vi "CH3_Save_Header.vi"() -> ()   [LabVIEW 2018]
uses:
  RxTx/RxTx.lvclass
  Save Image/Save Image.lvclass
panel:
  in  "Save Image out":refnum<class "Save Image.lvclass">
  in  "RxTx.lvclass":refnum<class "RxTx.lvclass">
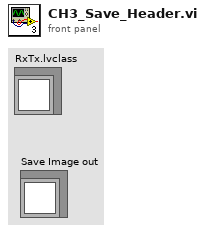
[diagram p1: front panel]
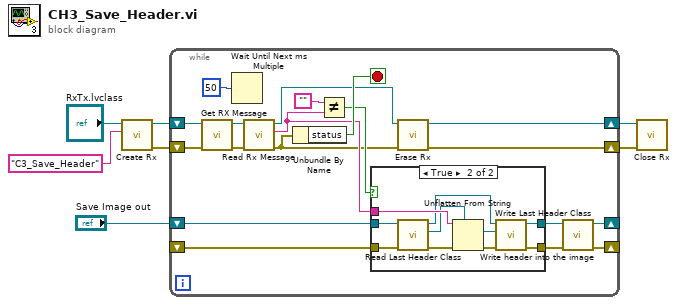
[diagram p0: block diagram]
diagram:
  n1 = call "Create Rx.vi"("Reader Name"="C3_Save_Header", "RxTx in"="RxTx.lvclass") -> ("error out"=w4:errorcluster, "RxTx out"=w5:refnum<class "RxTx.lvclass">)  [unwired: 8 in]
  n2 = while {
    shift-right: [w9] -> w2
    shift-left: w4 -> [w23]
    shift-right: [w10] -> w3
    shift-left: w5 -> [w24]
    shift-right: [w12] -> _
    shift-left: "Save Image out" -> [w14]
    shift-right: [w13] -> _
    shift-left: _ -> [w15]
    stop <- w25 stop-if-true
    n3 = call "Get RX Message.vi"("error in (no error)"=w23, "RxTx in"=w24) -> ("error out"=w21:errorcluster, "RxTx out"=w22:refnum<class "RxTx.lvclass">)  [unwired: 8 in]
    n4 = Wait Until Next ms Multiple(millisecond multiple=u32 50) -> ()  [unwired: 1 out]
    n5 = call "Read Rx Message.vi"("error in (no error)"=w21, "RxTx in"=w22) -> ("error out"=w8:errorcluster, "Rx Message"=w18:string, "RxTx out"=w11:refnum<class "RxTx.lvclass">)  [unwired: 7 in]
    n6 = Unbundle By Name(w8) -> ("status"=w25:bool)
    n7 = Not Equal?(x="", y=w18) -> (x != y?=w19:bool)
    n8 = case shown="True" w19 {
      tunnel: w18 -> [_ w38]
      tunnel: [w28 w29] -> w17
      tunnel: [w27 w30] -> w16
      tunnel: w15 -> [w27 w33]
      tunnel: w14 -> [w28 w34]
      frame False {
      }
      frame True {
        n9 = call "Read Last Header Class.vi"("error in (no error)"=w33, "Save Image in"=w34) -> ("error out"=w32:errorcluster, "Simulated_Header.lvclass"=w37:refnum<class "Simulated_Header.lvclass">, "Save Image out"=w35:refnum<class "Save Image.lvclass">)  [unwired: 7 in]
        n10 = Unflatten From String(type=w37, binary string=w38, error in (no error)=w32) -> (value=w36:refnum<class "Simulated_Header.lvclass">, error out=w31:errorcluster)  [unwired: 2 in, 1 out]
        n11 = call "Write Last Header Class.vi"("error in (no error)"=w31, "Simulated_Header.lvclass"=w36, "Save Image in"=w35) -> ("error out"=w30:errorcluster, "Save Image out"=w29:refnum<class "Save Image.lvclass">)  [unwired: 7 in]
      }
    }
    n12 = call "Erase Rx.vi"("error in (no error)"=w8, "RxTx in"=w11) -> ("error out"=w9:errorcluster, "RxTx out"=w10:refnum<class "RxTx.lvclass">)  [unwired: 8 in]
    n13 = call "Write header into the image.vi"("error in (no error)"=w16, "Save Image in"=w17) -> ("error out"=w13:errorcluster, "Save Image out"=w12:refnum<class "Save Image.lvclass">)  [unwired: 8 in]
  }
  n14 = call "Close Rx.vi"("error in (no error)"=w2, "RxTx in"=w3) -> ()  [unwired: 8 in, 2 out]
